vi "AutoSteerAngle.vi"(4 "CurrentSteerAngle":dbl, 6 "CurrentDirection":dbl, 8 "Ycurrent":dbl, 9 "Xcurrent":dbl, 10 "Ywaypoint":dbl, 11 "Xwaypoint":dbl) -> (2 "NewSteerAngle":dbl)   [LabVIEW 2012]
doc: "This VI calculates steering angle from current robot position to next waypoint."
uses:
  <vilib>/addons/control/pid/pid.llb/PID (DBL).vi
  <vilib>/addons/control/pid/NI_PID_pid.lvlib
panel:
  in  "reinitialize? (F)":bool
  out "reranged":dbl
  out "SetpointCommand":dbl
  out "Waveform Chart 2":cluster{dbl, dbl}(graph)
  out "output range":cluster{"output high":dbl, "output low":dbl}={"output high"=100.0, "output low"=-100.0} {"output low" format="%.2f"; "output high" format="%.2f"}
  out "PID gains":T1={"proportional gain (Kc)"=20.0, "integral time (Ti, min)"=0.008, "derivative time (Td, min)"=0.001} {"derivative time (Td, min)" step=1e-05 format="%.5f"; "integral time (Ti, min)" step=0.0001 format="%.4f"; "proportional gain (Kc)" step=0.001 format="%.4f"}
  out "Waveform Chart":cluster{dbl, "CurrentDirection":dbl}(graph)
  out "towaypoint":dbl
  # "This Vi calculates sttering angle \nfrom current position to \nnext waypoint"
  # "0.120\n1.600\n0000"
  # "in degreees"
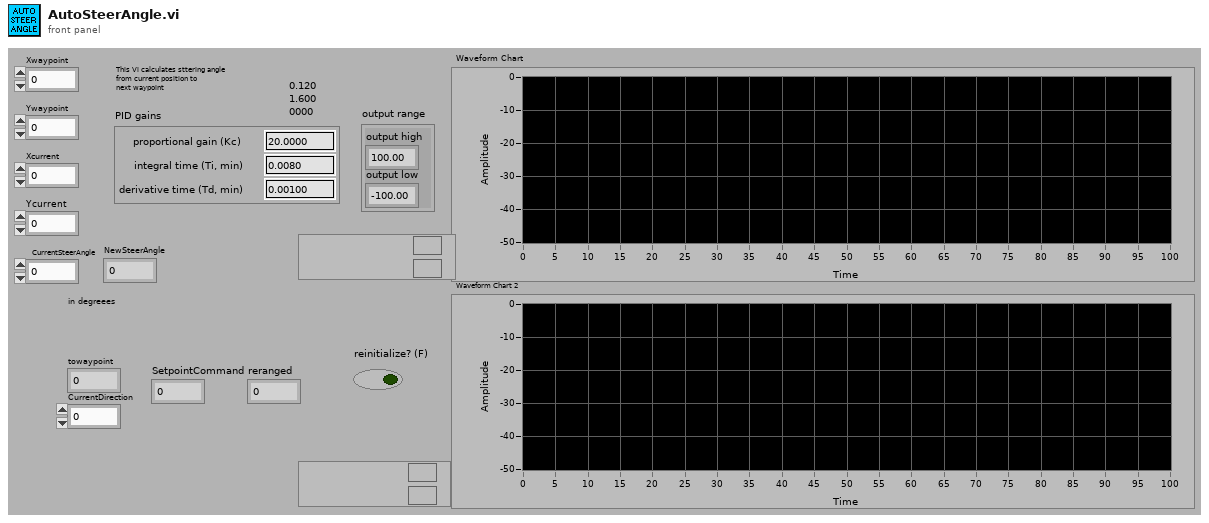
[diagram p1: front panel]
types:
  T1 = cluster{"proportional gain (Kc)":dbl, "integral time (Ti, min)":dbl, "derivative time (Td, min)":dbl}
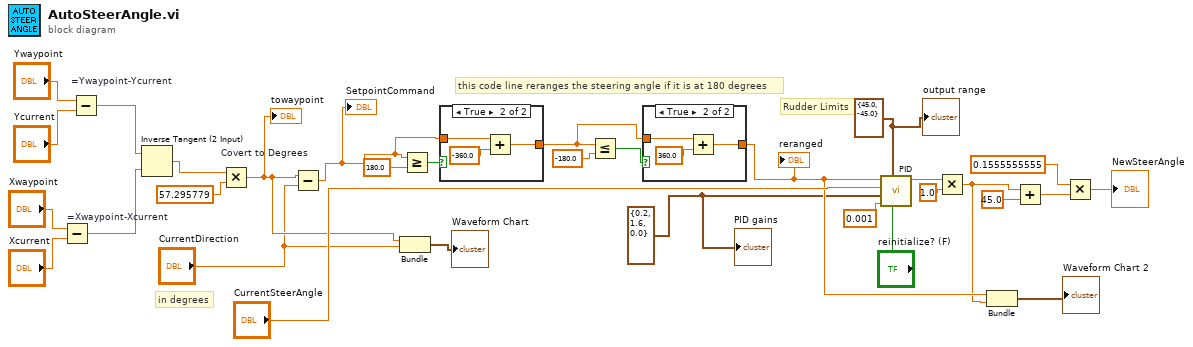
[diagram p0: block diagram]
diagram:
  w6 = T1 {"proportional gain (Kc)"=0.2, "integral time (Ti, min)"=1.6, "derivative time (Td, min)"=0.0} ("PID gains")
  w20 = cluster{"output high":dbl, "output low":dbl} {"output high"=45.0, "output low"=-45.0} ("output range")
  # "this code line reranges the steering angle if it is at 180 degrees"
  # "Rudder Limits"
  # "in degrees"
  n1 = Subtract "=Xwaypoint-Xcurrent"(x="Xwaypoint", y="Xcurrent") -> (x-y=w26:dbl)
  n2 = Subtract "=Ywaypoint-Ycurrent"(x="Ywaypoint", y="Ycurrent") -> (x-y=w27:dbl)
  n3 = Inverse Tangent (2 Input)(1:w26, 2:w27) -> (0:w24:dbl)
  n4 = Multiply "Covert to Degrees"(x=w24, y=57.295779) -> (x*y=w12:dbl)
  "towaypoint" <- w12
  n5 = Subtract(x=w12, y="CurrentDirection") -> (x-y=w16:dbl)
  "SetpointCommand" <- w16
  n6 = Bundle(w12, "CurrentDirection"="CurrentDirection") -> (→"Waveform Chart":cluster{dbl, "CurrentDirection":dbl})  [unwired: 1 in]
  n7 = Greater Or Equal?(x=w16, y=180.0) -> (x >= y?=w17:bool)
  n8 = case shown="True" w17 {
    tunnel: w16 -> [w32 w35]
    tunnel: [w32 w33] -> w13
    frame False {
    }
    frame True {
      n9 = Add(x=w35, y=-360.0) -> (x+y=w33:dbl)
    }
  }
  n10 = Less Or Equal?(x=w13, y=-180.0) -> (x <= y?=w14:bool)
  n11 = case shown="True" w14 {
    tunnel: w13 -> [w36 w39]
    tunnel: [w36 w37] -> w9
    frame False {
    }
    frame True {
      n12 = Add(x=w39, y=360.0) -> (x+y=w37:dbl)
    }
  }
  "reranged" <- w9
  n13 = call-poly <vilib>:"PID.vi"("reinitialize? (F)"="reinitialize? (F)", "output range"=w20, "dt (s)"=0.001, "PID gains"=w6, "process variable"="CurrentSteerAngle", "setpoint"=w9) -> ("output"=w21:dbl)  [unwired: 4 in, 1 out]
  n14 = Multiply(x=w21, y=1.0) -> (x*y=w4:dbl)
  n15 = Bundle(w9, w4) -> (→"Waveform Chart 2":cluster{dbl, dbl})  [unwired: 1 in]
  n16 = Add(x=w4, y=45.0) -> (x+y=w3:dbl)
  n17 = Multiply(x=0.1555555555, y=w3) -> (x*y=→"NewSteerAngle":dbl)
  "PID gains" <- w6
  "output range" <- w20
